vi "Transform xy.vi"(0 "y":dbl, 3 "x":dbl, 4 "2xN Matrix":T1=[[0.8660254037844387, -0.49999999999999994, 0.0], [0.49999999999999994, 0.8660254037844387, 0.0]]) -> (2 "y t":dbl, 5 "x t":dbl)   [LabVIEW 2023, in "Freetype Drawer.lvlib"]
uses:
  <vilib>/Analysis/Matrix/Datatypes/RealMatrix.ctl
  Freetype Drawer.lvlib
  <vilib>/Analysis/Matrix/NI_Matrix.lvlib
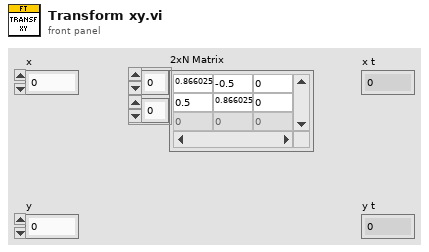
[diagram p1: front panel]
types:
  T1 = typedef "NI_Matrix.lvlib/RealMatrix.ctl" = dbl[][]
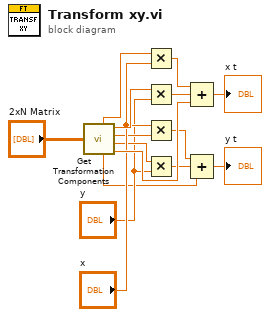
[diagram p0: block diagram]
diagram:
  n1 = call "Get Transformation Components.vi"("2xN Matrix"="2xN Matrix") -> ("xx"=w14:dbl, "ty"=w3:dbl, "xy"=w13:dbl, "yx"=w6:dbl, "yy"=w5:dbl, "tx"=w10:dbl)
  n2 = Multiply(x=w14, y="x") -> (x*y=w12:dbl)
  n3 = Multiply(x=w13, y="y") -> (x*y=w11:dbl)
  n4 = Multiply(x="x", y=w6) -> (x*y=w8:dbl)
  n5 = Multiply(x=w5, y="y") -> (x*y=w9:dbl)
  n6 = Compound Arithmetic op=ADD(w12, w11, w10) -> (→"x t":dbl)
  n7 = Compound Arithmetic op=ADD(w8, w9, w3) -> (→"y t":dbl)
